vi "Global Variabeln.vi"() -> ()   [LabVIEW 2021]
panel:
  in  "Humidity":dbl
  in  "Temperatur":dbl
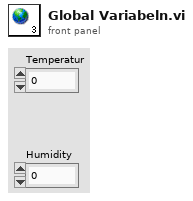
[diagram p1: front panel]
diagram:
